vi "Link to Bus.vi"(8 "error in (no error)":errorcluster, 10 "Fault-Injection Bus.lvclass":refnum<class "Fault-Injection Bus.lvclass">, 11 "Local Bus_DBL in":refnum<class "Fault-Injection_U32.lvclass">) -> (0 "error out":errorcluster, 3 "Local Bus_DBL out":refnum<class "Fault-Injection_U32.lvclass">)   [LabVIEW 2021, in "Fault-Injection_U32.lvclass"]
uses:
  Fault-Injection_U32.lvclass
  Fault-Injection_U32.lvclass/Fault-Injection_U32.ctl
  Fault-Injection Bus.lvclass
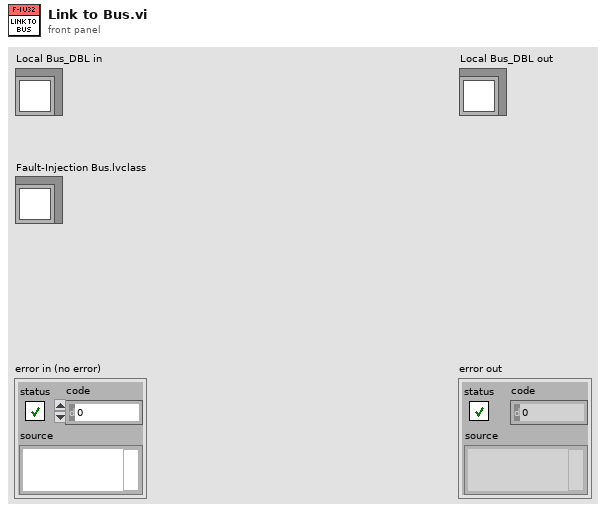
[diagram p1: front panel]
types:
  T1 = typedef "Fault-Injection Bus.lvclass/DVR Type.ctl" = cluster{"Boolean":refnum<data-value>, "String":refnum<data-value>, "DBL":refnum<data-value>, "SGL":refnum<data-value>, "EXT":refnum<data-value>, "U8":refnum<data-value>, "U16":refnum<data-value>, "U32":refnum<data-value>, "U64":refnum<data-value>, "I8":refnum<data-value>, "I16":refnum<data-value>, "I32":refnum<data-value>, "I64":refnum<data-value>, "CDBL":refnum<data-value>, "CSGL":refnum<data-value>, "CEXT":refnum<data-value>, "Time":refnum<data-value>, "Variant":refnum<data-value>, "Waveform":refnum<data-value>, "Type":refnum<data-value>}
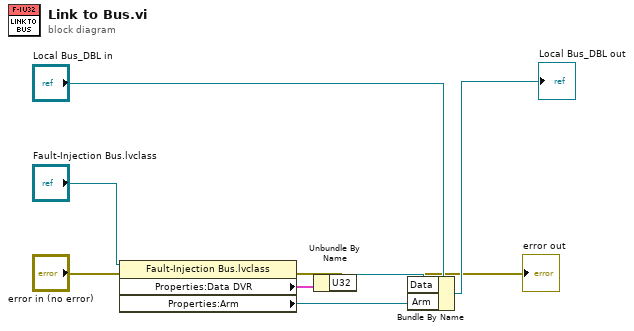
[diagram p0: block diagram]
diagram:
  n1 = property class="Fault-Injection Bus.lvclass"(reference="Fault-Injection Bus.lvclass", error in="error in (no error)") -> (error out=→"error out":errorcluster, "Properties:Data DVR"=w5:T1, "Properties:Arm"=w1:refnum<data-value>)  [unwired: 1 out]
  n2 = Unbundle By Name(w5) -> ("U32"=w4:refnum<data-value>)
  n3 = Bundle By Name(cluster="Local Bus_DBL in", "Data"=w4, "Arm"=w1) -> (→"Local Bus_DBL out":refnum<class "Fault-Injection_U32.lvclass">)
